vi "圆形分布指示灯（8）.vi"() -> ()   [LabVIEW 2012]
uses:
  <vilib>/Utility/miscctls.llb/LVBoundsTypeDef.ctl
  <vilib>/Analysis/1siggen.llb/Ramp Pattern by Samples.vi
  <vilib>/Analysis/NI_AALBase.lvlib
panel:
  in  "按钮大小":T1={"Width"=12, "Height"=12}
  in  "R":dbl=30.0
  out "Led7":bool=TRUE
  out "Led6":bool
  out "Led5":bool=TRUE
  out "Led4":bool
  out "Led3":bool
  out "Led2":bool
  out "Led1":bool
  out "Led0":bool
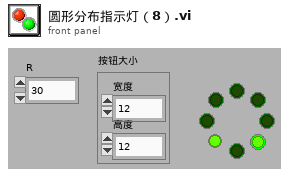
[diagram p1: front panel]
types:
  T1 = typedef "LVBoundsTypeDef.ctl" = cluster{"Width":u32, "Height":u32}
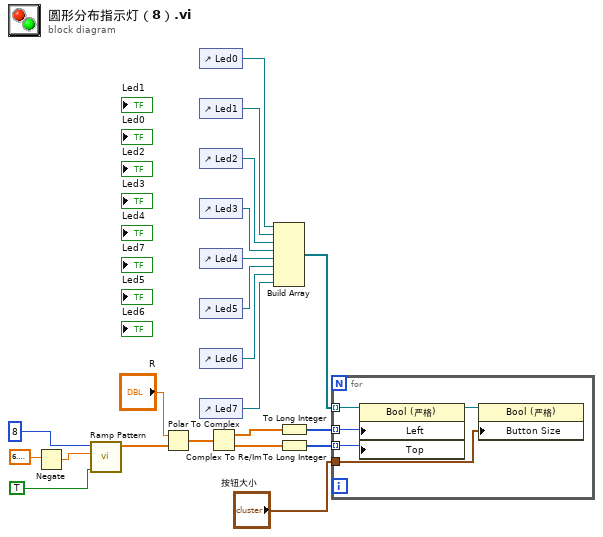
[diagram p0: block diagram]
diagram:
  n1 = Negate(x=6.283185307179586) -> (-x=w2:dbl)
  n2 = call-poly <vilib>:"Ramp Pattern.vi"("exclude end?"=TRUE, "end"=w2, "samples"=8) -> ("Ramp Pattern"=w12:dbl[])  [unwired: 7 in, 1 out]
  n3 = Polar To Complex(1:w12, 2:"R") -> (0:w11:cdb[])
  n4 = control-ref of="Led0"() -> (w21:refnum<vi>)
  n5 = control-ref of="Led1"() -> (w20:refnum<vi>)
  n6 = control-ref of="Led2"() -> (w19:refnum<vi>)
  n7 = control-ref of="Led3"() -> (w18:refnum<vi>)
  n8 = control-ref of="Led4"() -> (w17:refnum<vi>)
  n9 = control-ref of="Led5"() -> (w16:refnum<vi>)
  n10 = control-ref of="Led6"() -> (w15:refnum<vi>)
  n11 = control-ref of="Led7"() -> (w14:refnum<vi>)
  n12 = Complex To Re/Im(x + iy=w11) -> (x=w8:dbl[], y=w7:dbl[])
  n13 = Build Array(w21, w20, w19, w18, w17, w16, w15, w14) -> (w9:refnum<vi>[])
  n14 = To Long Integer(number=w8) -> (32bit integer=w6:i32[])
  n15 = To Long Integer(number=w7) -> (32bit integer=w5:i32[])
  n16 = for {
    tunnel: w9 -> [w26] mode=indexing
    tunnel: w6 -> [w25] mode=indexing
    tunnel: w5 -> [w24] mode=indexing
    tunnel: "按钮大小" -> [w22]
    n17 = property class="Bool (严格)"(reference=w26, "Left"=w25, "Top"=w24) -> (reference out=w23:refnum<vi>)  [unwired: 1 in, 1 out]
    n18 = property class="Bool (严格)"(reference=w23, "Button Size"=w22) -> ()  [unwired: 1 in, 2 out]
  }
